vi "5.2.vi"() -> ()   [LabVIEW 2017]
panel:
  out "任务二":string
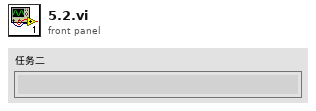
[diagram p1: front panel]
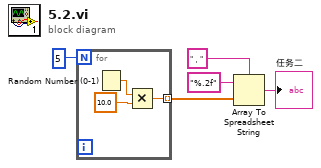
[diagram p0: block diagram]
diagram:
  n1 = for {
    N: 5 -> [_]
    tunnel: [w6] -> w4 mode=indexing
    n2 = Random Number (0-1)() -> (number: 0 to 1=w8:dbl)
    n3 = Multiply(x=w8, y=10.0) -> (x*y=w6:dbl)
  }
  n4 = Array To Spreadsheet String(delimiter (Tab)="，", array=w4, 3:"%.2f") -> (spreadsheet string=→"任务二":string)
